vi "Space & Group 2 Text.vi"(9 "Act Channel Group Type":T1, 10 "Cart Channel Group Type":T2, 11 "Space Group Type":T3) -> (2 "Text":string)   [LabVIEW 2013]
uses:
  Names/Space Group Type.ctl
  Names/Cart Channel  Group Type.ctl
  Names/Act Channel Group Type.ctl
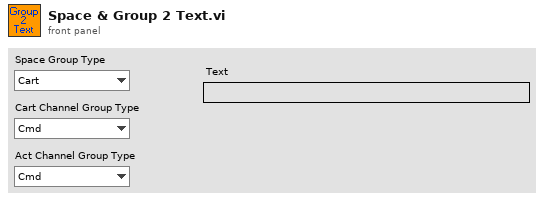
[diagram p1: front panel]
types:
  T1 = typedef "Act Channel Group Type.ctl" = enum16{"Cmd", "Disp", "Force", "ServoError"}
  T2 = typedef "Cart Channel  Group Type.ctl" = enum16{"Cmd", "Disp", "Load"}
  T3 = typedef "Space Group Type.ctl" = enum16{"Cart", "Act"}
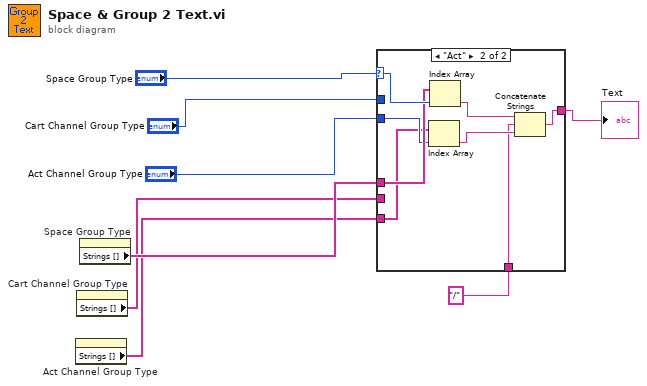
[diagram p0: block diagram]
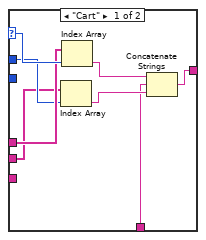
[diagram p2: hidden frame]
diagram:
  n1 = property on="Act Channel Group Type" class="Enum (strict)"() -> ("Strings []"=w3:string[])  [unwired: 2 in, 2 out]
  n2 = property on="Cart Channel Group Type" class="Enum (strict)"() -> ("Strings []"=w4:string[])  [unwired: 2 in, 2 out]
  n3 = property on="Space Group Type" class="Enum (strict)"() -> ("Strings []"=w5:string[])  [unwired: 2 in, 2 out]
  n4 = case shown="\"Act\"" "Space Group Type" {
    selector: "Space Group Type" -> [w16 w24]
    tunnel: "Cart Channel Group Type" -> [w14 _]
    tunnel: "Act Channel Group Type" -> [_ w18]
    tunnel: w5 -> [w15 w23]
    tunnel: w4 -> [w13 _]
    tunnel: w3 -> [_ w17]
    tunnel: "/" -> [w11 w21]
    tunnel: [w9 w19] -> w1
    frame "Cart" {
      n5 = Index Array(array=w13, index=w14) -> (element=w12:string)
      n6 = Index Array(array=w15, index=w16) -> (element=w10:string)
      n7 = Concatenate Strings(w10, w11, w12) -> (w9:string)
    }
    frame "Act" {
      n8 = Index Array(array=w17, index=w18) -> (element=w22:string)
      n9 = Index Array(array=w23, index=w24) -> (element=w20:string)
      n10 = Concatenate Strings(w20, w21, w22) -> (w19:string)
    }
  }
  "Text" <- w1
